vi "G-Unicode UTF-8 Class Editor.vi"(6 "Variant in":variant, 7 "Shift Pressed?":bool, 8 "error in (no error)":errorcluster, 10 "QD Combo Box Ref":refnum<vi>, 11 "QD Launch VI Ref":refnum<vi>) -> (0 "error out":errorcluster, 4 "Variant out":variant)   [LabVIEW 2020]
doc: "View and edit a UTF-8 String or UTF-8 Path class value.\n\nDefault Shortcut - [G]"
uses:
  Types/UTF-8 String/UTF-8 String.lvclass
  Types/UTF-8 Path/UTF-8 Path.lvclass
  Types/UTF-8 Path/UTF-8 Path.lvclass/UTF-8 Path.ctl
  Types/UTF-8 String/UTF-8 String.lvclass/UTF-8 String.ctl
  5c5e70dc-6712-4b74-bcca-18931564a8c0.vi
  Private/Conversion/String as Encoded String.vi
  Private/Conversion/Polymorphic VIs/String as Encoded String (LabVIEW String).vi
  Private/Conversion/Polymorphic VIs/String as Encoded String (UTF-8 String).vi
  Private/Conversion/Text to UTF-8.vi
  Private/Conversion/Polymorphic VIs/Text to UTF-8 (LabVIEW String).vi
  Private/Library/gu_input_box.vi
panel:
  in  "Undo Name":string="Edit UTF-8 Value"
  # "Do not change the connector pane of this VI.\n\nSee the block diagram for directions on how to use this template."
  # "Specify the name of the Undo transaction"
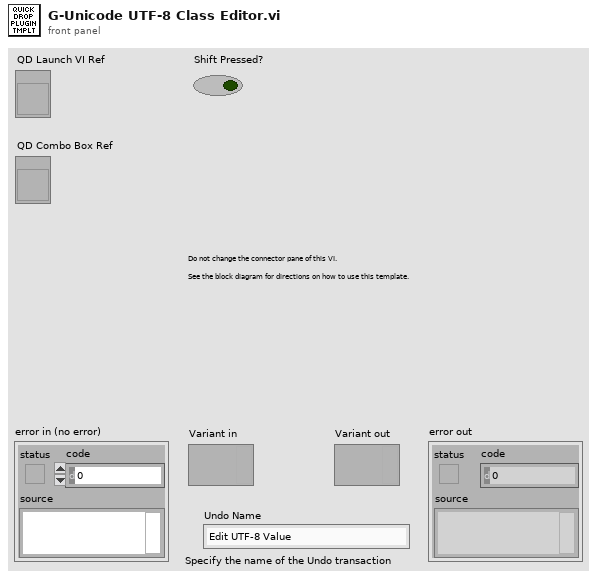
[diagram p1: front panel]
types:
  T1 = typedef "G-Unicode.lvlib/Encoded UTF-8 Path.ctl" = path
  T2 = enum16{"UTF-8 String", "UTF-8 Path", "Unknown"}[]
  T3 = typedef "G-Unicode.lvlib/Encoded UTF-8 String.ctl" = string
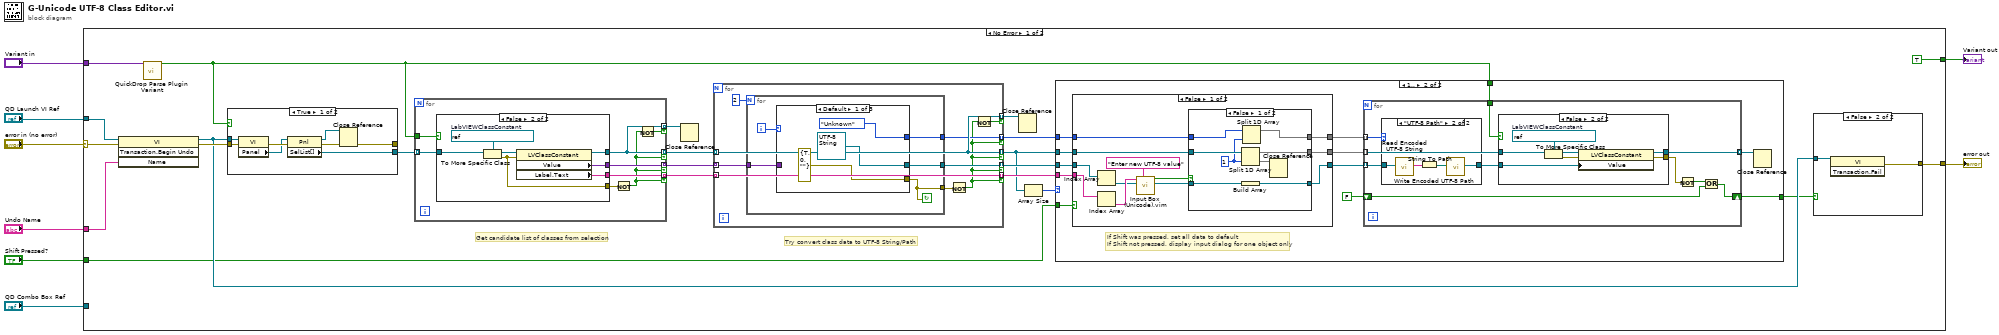
[diagram p0: block diagram]
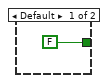
[diagram p2: hidden frame]
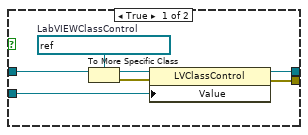
[diagram p4: hidden frame]
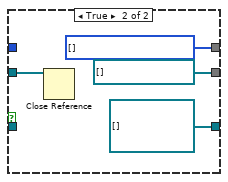
[diagram p5: hidden frame]
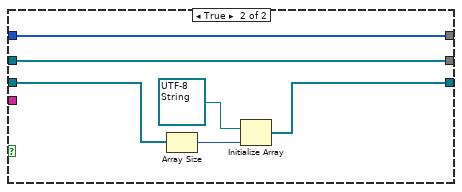
[diagram p6: hidden frame]
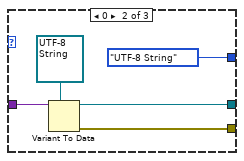
[diagram p7: hidden frame]
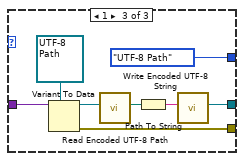
[diagram p8: hidden frame]
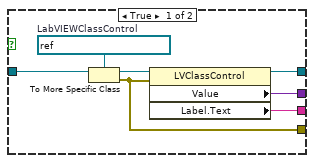
[diagram p9: hidden frame]
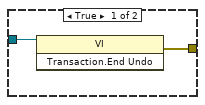
[diagram p10: hidden frame]
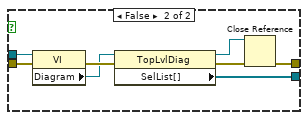
[diagram p11: hidden frame]
diagram:
  n1 = case shown="No Error" "error in (no error)" {
    selector: "error in (no error)" -> [w29 w175]
    tunnel: [w24 w175] -> w7
    tunnel: "QD Launch VI Ref" -> [w28 _]
    tunnel: "Shift Pressed?" -> [w12 _]
    tunnel: "QD Combo Box Ref" -> [_ _]
    tunnel: "Variant in" -> [w30 _]
    tunnel: "Undo Name" -> [w27 _]
    tunnel: [TRUE _] -> w1
    frame No Error {
      # "Try convert class data to UTF-8 String/Path"
      # "Get candidate list of classes from selection"
      n2 = invoke class="VI" method="Transaction.Begin Undo"(reference=w28, error in=w29, "Name"=w27) -> (reference out=w23:refnum<vi>, error out=w25:errorcluster)  [unwired: 1 in, 2 out]
      n3 = call <vilib>:"QuickDrop Parse Plugin Variant.vi"("QDKS Variant in"=w30) -> ("QD Launch VI Panel?"=w13:bool)  [unwired: 12 in, 2 out]
      n4 = case shown="True" w13 {
        tunnel: w25 -> [w166 w174]
        tunnel: w23 -> [w165 w173]
        tunnel: [w160 w168] -> _
        tunnel: [w159 w167] -> w14
        frame True {
          n5 = property class="VI"(reference=w165, error in=w166) -> (error out=w164:errorcluster, "Panel"=w163:refnum<vi>)  [unwired: 1 out]
          n6 = property class="Pnl"(reference=w163, error in=w164) -> (reference out=w161:refnum<vi>, error out=w162:errorcluster, "SelList[]"=w159:refnum<vi>[])
          n7 = Close Reference(reference=w161, error in (no error)=w162) -> (error out=w160:errorcluster)
        }
        frame False {
          n8 = property class="VI"(reference=w173, error in=w174) -> (error out=w172:errorcluster, "Diagram"=w171:refnum<vi>)  [unwired: 1 out]
          n9 = property class="TopLvlDiag"(reference=w171, error in=w172) -> (reference out=w169:refnum<vi>, error out=w170:errorcluster, "SelList[]"=w167:refnum<vi>[])
          n10 = Close Reference(reference=w169, error in (no error)=w170) -> (error out=w168:errorcluster)
        }
      }
      n11 = for {
        tunnel: [w140] -> w15 mode=indexing if=w135
        tunnel: [w139] -> w16 mode=indexing if=w135
        tunnel: w14 -> [w138] mode=indexing
        tunnel: [w136] -> w18 mode=indexing if=w135
        tunnel: [w136] -> w17 mode=indexing if=w134
        tunnel: w13 -> [w133]
        n12 = case shown="False" w133 {
          tunnel: [w145 w152] -> w140
          tunnel: [w144 w151] -> w139
          tunnel: w138 -> [w143 w150]
          tunnel: [w142 w149] -> w136
          tunnel: [w141 w148] -> w137
          frame True {
            w146 = refnum<vi> refnum  # LabVIEWClassControl
            n13 = To More Specific Class(target class=w146, reference=w143) -> (specific class reference=w147:refnum<vi>, error out=w141:errorcluster)  [unwired: 1 in]
            n14 = property class="LVClassControl"(reference=w147, error in=w141) -> (reference out=w142:refnum<vi>, "Value"=w145:variant, "Label.Text"=w144:string)  [unwired: 1 out]
          }
          frame False {
            w153 = refnum<vi> refnum  # LabVIEWClassConstant
            n15 = To More Specific Class(target class=w153, reference=w150) -> (specific class reference=w154:refnum<vi>, error out=w148:errorcluster)  [unwired: 1 in]
            n16 = property class="LVClassConstant"(reference=w154, error in=w148) -> (reference out=w149:refnum<vi>, "Value"=w152:variant, "Label.Text"=w151:string)  [unwired: 1 out]
          }
        }
        n17 = Not(x=w137) -> (.not. x?=w135:bool)
        n18 = Not(x=w135) -> (.not. x?=w134:bool)
      }
      n19 = Close Reference(reference=w17) -> ()  [unwired: 1 in, 1 out]
      n20 = for {
        tunnel: w15 -> [w110] mode=indexing
        tunnel: w16 -> [w107] mode=indexing
        tunnel: w18 -> [w106] mode=indexing
        tunnel: [w109] -> w20 mode=indexing if=w103
        tunnel: [w106] -> w10 mode=indexing if=w103
        tunnel: [w107] -> w21 mode=indexing if=w103
        tunnel: [w106] -> w19 mode=indexing if=w105
        tunnel: [w104] -> w22 mode=indexing if=w103
        n21 = for {
          N: 2 -> [_]
          tunnel: w110 -> [w115]
          tunnel: [w114] -> w109
          tunnel: [w113] -> w108
          tunnel: [w112] -> w104
          i -> [w116]
          stop <- w113 continue-if-true
          n22 = case shown="Default" w116 {
            tunnel: w115 -> [_ w123 w131]
            tunnel: [refnum<class "UTF-8 String.lvclass"> refnum ("UTF-8 String") w122 w127] -> w114
            tunnel: [errorcluster {"status"=TRUE, "code"=0, "source"=""} ("error out") w121 w130] -> w113
            tunnel: [enum16{"UTF-8 String", "UTF-8 Path", "Unknown"}."Unknown" enum16{"UTF-8 String", "UTF-8 Path", "Unknown"}."UTF-8 String" enum16{"UTF-8 String", "UTF-8 Path", "Unknown"}."UTF-8 Path"] -> w112
            frame Default {
            }
            frame 0 {
              n23 = Variant To Data(type=refnum<class "UTF-8 String.lvclass"> refnum ("G-Unicode.lvlib:UTF-8 String.lvclass"), Variant=w123) -> (data=w122:refnum<class "UTF-8 String.lvclass">, error out=w121:errorcluster)  [unwired: 1 in]
            }
            frame 1 {
              n24 = Variant To Data(type=refnum<class "UTF-8 Path.lvclass"> refnum ("G-Unicode.lvlib:UTF-8 Path.lvclass"), Variant=w131) -> (data=w129:refnum<class "UTF-8 Path.lvclass">, error out=w130:errorcluster)  [unwired: 1 in]
              n25 = call "Read Encoded UTF-8 Path.vi"("UTF-8 Path"=w129) -> ("Encoded UTF-8 Path"=w128:T1)  [unwired: 10 in]
              n26 = Path To String(path=w128) -> (string=w126:string)
              n27 = call "Write Encoded UTF-8 String.vi"("Encoded UTF-8 String"=w126) -> ("UTF-8 String"=w127:refnum<class "UTF-8 String.lvclass">)  [unwired: 10 in]
            }
          }
        }
        n28 = Not(x=w108) -> (.not. x?=w103:bool)
        n29 = Not(x=w103) -> (.not. x?=w105:bool)
      }
      n30 = Close Reference(reference=w19) -> ()  [unwired: 1 in, 1 out]
      n31 = Array Size(array=w10) -> (size(s)=w9:i32)
      n32 = case shown="1.." w9 {
        tunnel: w22 -> [_ w41]
        tunnel: w21 -> [_ w37]
        tunnel: w20 -> [_ w36]
        tunnel: w10 -> [_ w35]
        tunnel: w13 -> [_ w34]
        tunnel: w12 -> [_ w33]
        tunnel: [FALSE w32] -> w11
        frame Default {
        }
        frame 1.. {
          # "If Shift was pressed, set all data to default\nIf Shift not pressed, display input dialog for one object only"
          n33 = case shown="False" w33 {
            tunnel: w35 -> [w84 w98]
            tunnel: w36 -> [w83 w102]
            tunnel: w37 -> [w82 _]
            tunnel: [w75 w99] -> w39
            tunnel: [w78 w98] -> w38
            tunnel: [w73 w97] -> w42
            tunnel: w41 -> [w74 w97]
            frame False {
              n34 = Index Array(array=w83) -> (element=w80:refnum<class "UTF-8 String.lvclass">)  [unwired: 1 in]
              n35 = Index Array(array=w82) -> (element=w81:string)  [unwired: 1 in]
              n36 = call "Input Box (Unicode).vim"("Prompt"="Enter new UTF-8 value", "Default Input"=w80, "Message"=w81) -> ("Input"=w76:refnum<class "UTF-8 String.lvclass">, "Cancelled"=w77:bool)  [unwired: 6 in, 1 out]
              n37 = case shown="False" w77 {
                tunnel: w84 -> [w92 w94]
                tunnel: [w90 refnum<vi>[] []] -> w78
                tunnel: w76 -> [w89 _]
                tunnel: [w88 refnum<class "UTF-8 String.lvclass">[] []] -> w75
                tunnel: w74 -> [w87 _]
                tunnel: [w85 w93] -> w73
                frame False {
                  w86 = 1 ("index")
                  n38 = Split 1D Array(array=w92, index=w86) -> (first subarray=w90:refnum<vi>[], second subarray=w91:refnum<vi>[])
                  n39 = Build Array(w89) -> (w88:refnum<class "UTF-8 String.lvclass">[])
                  n40 = Split 1D Array(array=w87, index=w86) -> (first subarray=w85:T2)  [unwired: 1 out]
                  n41 = Close Reference(reference=w91) -> ()  [unwired: 1 in, 1 out]
                }
                frame True {
                  w93 = T2 [] items=["UTF-8 String", "UTF-8 Path", "Unknown"]
                  n42 = Close Reference(reference=w94) -> ()  [unwired: 1 in, 1 out]
                }
              }
            }
            frame True {
              n43 = Array Size(array=w102) -> (size(s)=w101:i32)
              n44 = Initialize Array(refnum<class "UTF-8 String.lvclass"> refnum ("G-Unicode.lvlib:UTF-8 String.lvclass"), w101) -> (w99:refnum<class "UTF-8 String.lvclass">[])
            }
          }
          n45 = for {
            tunnel: w38 -> [w53] mode=indexing
            tunnel: w39 -> [w49] mode=indexing
            tunnel: [w52] -> w40 mode=indexing
            tunnel: w42 -> [w51] mode=indexing
            shift-right: [w45] -> w32
            shift-left: FALSE -> [w46]
            tunnel: w34 -> [w44]
            n46 = case shown="\"UTF-8 Path\"" w51 {
              tunnel: [w54 w55] -> w50
              tunnel: w49 -> [w54 w58]
              frame "UTF-8 String", Default {
              }
              frame "UTF-8 Path" {
                n47 = call "Read Encoded UTF-8 String.vi"("UTF-8 String"=w58) -> ("Encoded UTF-8 String"=w57:T3)  [unwired: 10 in]
                n48 = String To Path(string=w57) -> (path=w56:path)
                n49 = call "Write Encoded UTF-8 Path.vi"("Encoded UTF-8 Path"=w56) -> ("UTF-8 Path"=w55:refnum<class "UTF-8 Path.lvclass">)  [unwired: 10 in]
              }
            }
            n50 = case shown="False" w44 {
              tunnel: w53 -> [w63 w70]
              tunnel: [w62 w69] -> w52
              tunnel: w50 -> [w60 w67]
              tunnel: [w59 w66] -> w48
              frame True {
                w64 = refnum<vi> refnum  # LabVIEWClassControl
                n51 = To More Specific Class(target class=w64, reference=w63) -> (specific class reference=w65:refnum<vi>, error out=w61:errorcluster)  [unwired: 1 in]
                n52 = property class="LVClassControl"(reference=w65, error in=w61, "Value"=w60) -> (reference out=w62:refnum<vi>, error out=w59:errorcluster)
              }
              frame False {
                w71 = refnum<vi> refnum  # LabVIEWClassConstant
                n53 = To More Specific Class(target class=w71, reference=w70) -> (specific class reference=w72:refnum<vi>, error out=w68:errorcluster)  [unwired: 1 in]
                n54 = property class="LVClassConstant"(reference=w72, error in=w68, "Value"=w67) -> (reference out=w69:refnum<vi>, error out=w66:errorcluster)
              }
            }
            n55 = Not(x=w48) -> (.not. x?=w47:bool)
            n56 = Or(x=w47, y=w46) -> (x .or. y?=w45:bool)
          }
          n57 = Close Reference(reference=w40) -> ()  [unwired: 1 in, 1 out]
        }
      }
      n58 = case shown="False" w11 {
        tunnel: w23 -> [w155 w157]
        tunnel: [w156 w158] -> w24
        frame True {
          n59 = invoke class="VI" method="Transaction.End Undo"(reference=w155) -> (error out=w156:errorcluster)  [unwired: 2 in, 2 out]
        }
        frame False {
          n60 = invoke class="VI" method="Transaction.Fail"(reference=w157) -> (error out=w158:errorcluster)  [unwired: 2 in, 2 out]
        }
      }
    }
    frame Error {
    }
  }
  "error out" <- w7
  "Variant out" <- w1
